vi "Feedback Evaporative Cooler Demo.vi"() -> ()   [LabVIEW 2012]
uses:
  Cooler/Cooler/Cooler.lvclass
  Cooler UI/Cooler Panel/Cooler Panel.lvclass
  <vilib>/ActorFramework/Message Queue/Message Queue.lvclass/Message Queue.ctl
  Cooler UI/Write Cooler Msg/Write Cooler Msg.lvclass/Write Cooler Msg.ctl
  <vilib>/ActorFramework/Message Enqueuer/Message Enqueuer.lvclass/Message Enqueuer.ctl
  Cooler/Write UI Msg/Write UI Msg.lvclass/Write UI Msg.ctl
  <vilib>/ActorFramework/Message Enqueuer/Enqueue.vi
  <vilib>/ActorFramework/Message Priority Queue/Priority Enqueue.vi
  Cooler UI/Write Cooler Msg/Write Cooler Msg.lvclass
  Cooler/Write UI Msg/Write UI Msg.lvclass
  <vilib>/ActorFramework/Stop Msg/Stop Msg.lvclass
  <vilib>/ActorFramework/Actor/Actor.lvclass
  <vilib>/ActorFramework/Message Queue/Message Queue.lvclass
  Level Controller/Level Controller/Level Controller.lvclass
panel:
  in  "stop":bool
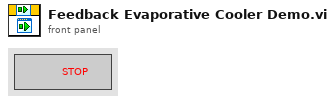
[diagram p1: front panel]
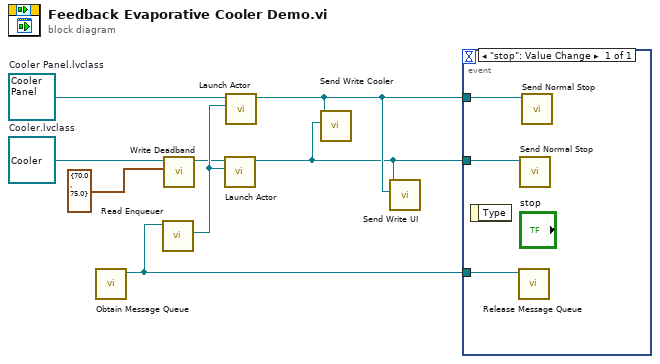
[diagram p0: block diagram]
diagram:
  w7 = refnum<class "Cooler Panel.lvclass"> refnum  # Cooler Panel.lvclass
  w3 = refnum<class "Cooler.lvclass"> refnum  # Cooler.lvclass
  n1 = call <vilib>:"Obtain Message Queue.vi"() -> ("Message Queue"=w8:refnum<class "Message Queue.lvclass">)  [unwired: 10 in, 1 out]
  n2 = call <vilib>:"Read Enqueuer.vi"("Message Queue"=w8) -> ("Message Enqueuer"=w6:refnum<class "Message Enqueuer.lvclass">)  [unwired: 10 in]
  n3 = call "Write Deadband.vi"("Deadband"=cluster{"LO":dbl, "HI":dbl} {"LO"=70.0, "HI"=75.0}, "Level Controller in"=w3) -> ("Level Controller out"=w2:refnum<class "Cooler.lvclass">)  [unwired: 8 in, 1 out]
  n4 = call <vilib>:"Launch Actor.vi"("Actor-to-Caller Enqueuer"=w6, "Actor"=w2) -> ("Caller-To-Actor Enqueuer"=w4:refnum<class "Message Enqueuer.lvclass">)  [unwired: 8 in, 1 out]
  n5 = call <vilib>:"Launch Actor.vi"("Actor-to-Caller Enqueuer"=w6, "Actor"=w7) -> ("Caller-To-Actor Enqueuer"=w5:refnum<class "Message Enqueuer.lvclass">)  [unwired: 8 in, 1 out]
  n6 = call "Send Write Cooler.vi"("Cooler"=w4, "enqueuer"=w5) -> ()  [unwired: 9 in, 1 out]
  n7 = call "Send Write UI.vi"("UI Queue"=w5, "enqueuer"=w4) -> ()  [unwired: 9 in, 1 out]
  n8 = event shown="[0] \"stop\": Value Change" {
    selector: _ -> [_]
    dyn-events: _ -> [_]
    timeout: _ -> [_]
    tunnel: w4 -> [w11]
    tunnel: w8 -> [w10]
    tunnel: w5 -> [w9]
    event "stop": Value Change {
      n9 = event-data() -> ()  [unwired: 1 in, 1 out]
      n10 = call <vilib>:"Release Message Queue.vi"("Message Queue"=w10) -> ()  [unwired: 9 in, 2 out]
      n11 = call <vilib>:"Send Normal Stop.vi"("Message Enqueuer"=w11) -> ()  [unwired: 10 in, 1 out]
      n12 = call <vilib>:"Send Normal Stop.vi"("Message Enqueuer"=w9) -> ()  [unwired: 10 in, 1 out]
    }
  }
